vi "Time FGV.vi"(7 "Set/Get":enum16{"Get", "Set"}(ring), 8 "error in (no error)":errorcluster, 10 "Target":dbl, 11 "Elevator Controller Actor in":refnum<class "Elevator Controller Actor.lvclass">) -> (0 "error out":errorcluster, 2 "Elapsed time":dbl, 3 "Elevator Controller Actor out":refnum<class "Elevator Controller Actor.lvclass">)   [LabVIEW 2022 SP3, in "Elevator Controller Actor.lvlib" / "Elevator Controller Actor.lvclass"]
uses:
  Elevator Controller Actor.lvclass
  Elevator Controller Actor.lvclass/Elevator Controller Actor.ctl
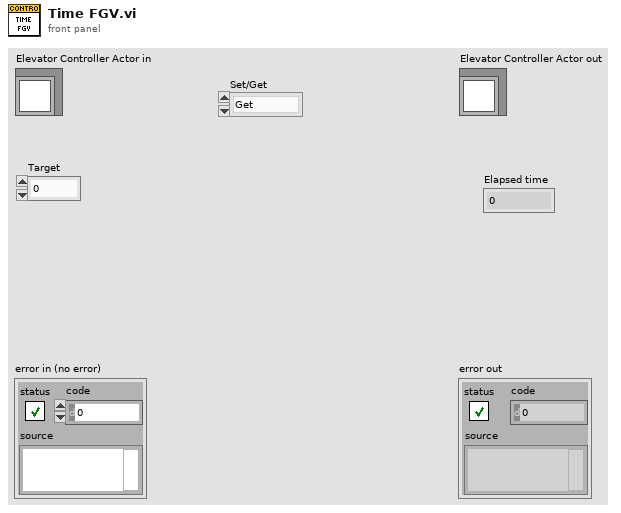
[diagram p1: front panel]
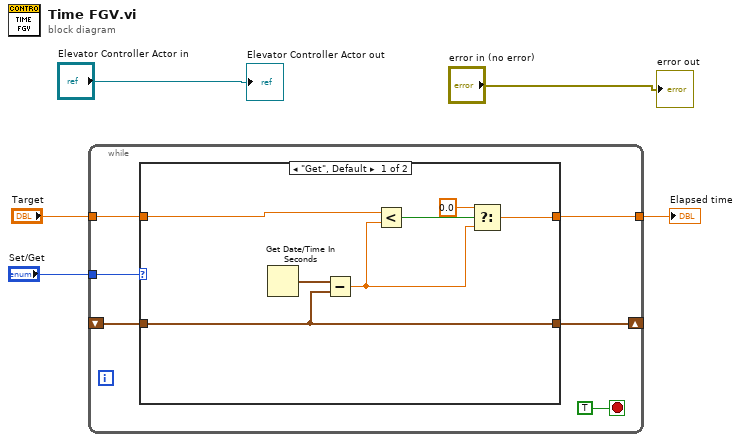
[diagram p0: block diagram]
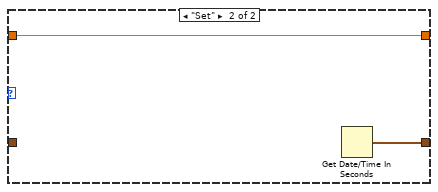
[diagram p2: hidden frame]
diagram:
  n1 = while {
    tunnel: "Set/Get" -> [w11]
    shift-right: [w8] -> _
    shift-left: _ -> [w10]
    tunnel: "Target" -> [w6]
    tunnel: [w7] -> w2
    stop <- TRUE stop-if-true
    n2 = case shown="\"Get\", Default" w11 {
      tunnel: w10 -> [w17 _]
      tunnel: [w17 w20] -> w8
      tunnel: [w12 w19] -> w7
      tunnel: w6 -> [w16 w19]
      frame "Get", Default {
        n3 = Get Date/Time In Seconds() -> (seconds since 1Jan1904=w18:timestamp)
        n4 = Subtract(x=w18, y=w17) -> (x-y=w14:dbl)
        n5 = Less?(x=w16, y=w14) -> (x < y?=w15:bool)
        n6 = Select(t=0.0, s=w15, f=w14) -> (s? t:f=w12:dbl)
      }
      frame "Set" {
        n7 = Get Date/Time In Seconds() -> (seconds since 1Jan1904=w20:timestamp)
      }
    }
  }
  "Elapsed time" <- w2
  "error out" <- "error in (no error)"
  "Elevator Controller Actor out" <- "Elevator Controller Actor in"
